vi "Select File.vi"(8 "error in (no error)":errorcluster, 10 "File Path":path, 11 "Data Loader in":refnum<class "Data Loader.lvclass">) -> (0 "error out":errorcluster, 3 "Data Loader out":refnum<class "Data Loader.lvclass">)   [LabVIEW 2020, in "Data Loader.lvlib" / "Data Loader.lvclass"]
uses:
  Data Loader.lvclass
  Data Loader.lvclass/Data Loader.ctl
  Depden On/MVVM Framework/MVVM Abstruct Model/MVVM Abstruct Model/MVVM Abstruct Model.lvclass/MVVM Abstruct Model.ctl
  Data Types/Abstrut Data/Abstruct Data Type.lvclass/Abstruct Data Type.ctl
  Views/Data List Infor Interface Messages/Data List Msg/Data List Msg.lvclass/Data List Msg.ctl
  <vilib>/ActorFramework/Message Enqueuer/Message Enqueuer.lvclass/Message Enqueuer.ctl
  Depden On/MVVM Framework/MVVM Abstruct Model/MVVM Abstruct Model/Accessor/Read ActorMap-Views.vi
  Data Types/Abstrut Data/Accessors/Read Table Infor.vi
  <vilib>/ActorFramework/Message Enqueuer/Enqueue.vi
  Views/Data List Infor Interface Messages/Data List Msg/Data List Msg.lvclass
  C:/Program Files (x86)/National Instruments/LabVIEW 2020/vi.lib/ActorFramework/Message/Message.lvclass
  <vilib>/ActorFramework/Message Priority Queue/Priority Enqueue.vi
  Depden On/ActorMap/ActorMap.lvclass
  Data List/Data List.lvclass
  Data Types/Abstrut Data/Abstruct Data Type.lvclass
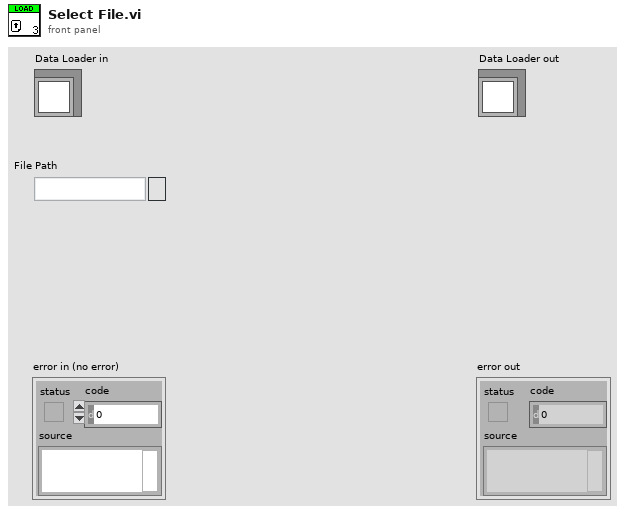
[diagram p1: front panel]
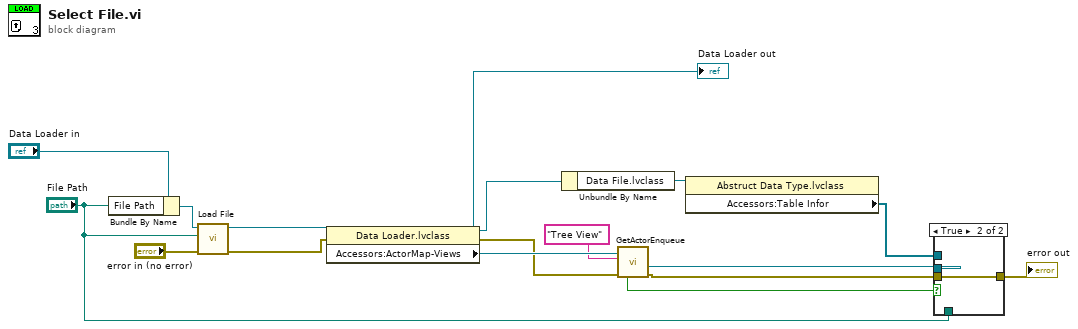
[diagram p0: block diagram]
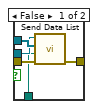
[diagram p2: hidden frame]
diagram:
  n1 = Bundle By Name(cluster="Data Loader in", "File Path"="File Path") -> (w15:refnum<class "Data Loader.lvclass">)
  n2 = call-dynamic "Load File.vi"("error in (no error)"="error in (no error)", "File Path"="File Path", "Data Loader in"=w15) -> ("error out"=w7:errorcluster, "Data Loader out"=w13:refnum<class "Data Loader.lvclass">)  [unwired: 7 in]
  n3 = property class="Data Loader.lvclass"(reference=w13, error in=w7) -> (reference out=w6:refnum<class "Data Loader.lvclass">, error out=w8:errorcluster, "Accessors:ActorMap-Views"=w12:refnum<class "ActorMap.lvclass">)
  "Data Loader out" <- w6
  n4 = Unbundle By Name(w6) -> ("Data File.lvclass"=w5:refnum<class "Abstruct Data Type.lvclass">)
  n5 = call "GetActorEnqueue.vi"("error in (no error)"=w8, "name"="Tree View", "ActorMap in"=w12) -> ("error out"=w2:errorcluster, "Enqueue"=w9:refnum<class "Message Enqueuer.lvclass">, "key not found?"=w10:bool)  [unwired: 5 in, 1 out]
  n6 = property class="Abstruct Data Type.lvclass"(reference=w5) -> ("Accessors:Table Infor"=w4:refnum<class "Data List.lvclass">[])  [unwired: 1 in, 2 out]
  n7 = case shown="True" w10 {
    tunnel: w9 -> [w20 _]
    tunnel: w4 -> [w21 _]
    tunnel: [w19 w22] -> w3
    tunnel: w2 -> [w18 w22]
    tunnel: "File Path" -> [w17 _]
    frame False {
      n8 = call "Send Data List.vi"("error in (no error)"=w18, "File Path"=w17, "Table Infor"=w21, "Message Enqueuer"=w20) -> ("error out"=w19:errorcluster)  [unwired: 6 in, 1 out]
    }
    frame True {
    }
  }
  "error out" <- w3
